vi "题目2.vi"() -> ()   [LabVIEW 2017]
panel:
  out "数值 2":i32
  out "数值":i32
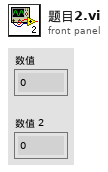
[diagram p1: front panel]
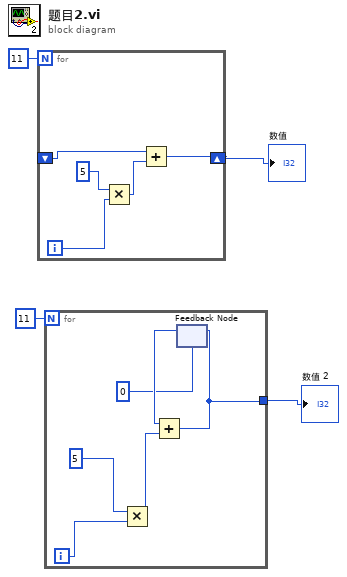
[diagram p0: block diagram]
diagram:
  n1 = for {
    N: 11 -> [_]
    shift-right: [w6] -> w2
    shift-left: _ -> [w5]
    i -> [w9]
    n2 = Multiply(x=5, y=w9) -> (x*y=w7:i32)
    n3 = Add(x=w5, y=w7) -> (x+y=w6:i32)
  }
  "数值" <- w2
  n4 = for {
    N: 11 -> [_]
    tunnel: [w12] -> w1
    i -> [w15]
    n5 = Multiply(x=5, y=w15) -> (x*y=w13:i32)
    n6 = feedback #1(0) -> (w11:i32)
    n7 = Add(x=w11, y=w13) -> (x+y=w12:i32)
    n8 = feedback-in #1(w12) -> ()
  }
  "数值 2" <- w1
